vi "Convert to Waveforms.vi"(0 "data in":sgl[][](array[numeric]) format="%#.21g", 1 "physical channels":T1[](array[typedef])=[enum."Voltage Phase A (L1)", enum."Voltage Phase B (L2)", enum."Voltage Phase C (L3)", enum."Current Phase A (L1)", enum."Current Phase B (L2)", enum."Current Phase C (L3)", enum."Current Phase N (Neutral)"], 2 "reset? (F)":bool, 5 "sample rate [Hz]":sgl=9600.0 format="%#.6g", 7 "timestamp":timestamp, 9 "system info in":refnum<class "EP System Info.lvclass">, 11 "error in (no error)":errorcluster) -> (4 "voltage waveforms":waveform(dbl)[](array[waveform]), 6 "current waveforms":waveform(dbl)[](array[waveform]), 10 "system info out":refnum<class "EP System Info.lvclass">, 14 "interval length [s]":dbl, 15 "error out":errorcluster)   [LabVIEW 2014, in "NI_EP_Power Quality.lvlib"]
doc: "Converts resampled voltage and current data to voltage and current waveforms of different line configurations. This VI also arranges the order of the elements in the waveforms of each three-phase electrical power system for further measurement. For example, the orders are A-B-C-N for the four-channel method and A-B-C for the three-channel method. You must manually select the polymorphic instance you want to use."
uses:
  <vilib>/addons/Electrical Power/PQ/NI_EP_Power Quality.lvlib
  <vilib>/addons/Electrical Power/PQ/Common/Classes/System Info/EP System Info.lvclass
  <vilib>/addons/Electrical Power/PQ/Common/Controls/ep_AI Data Channel.ctl
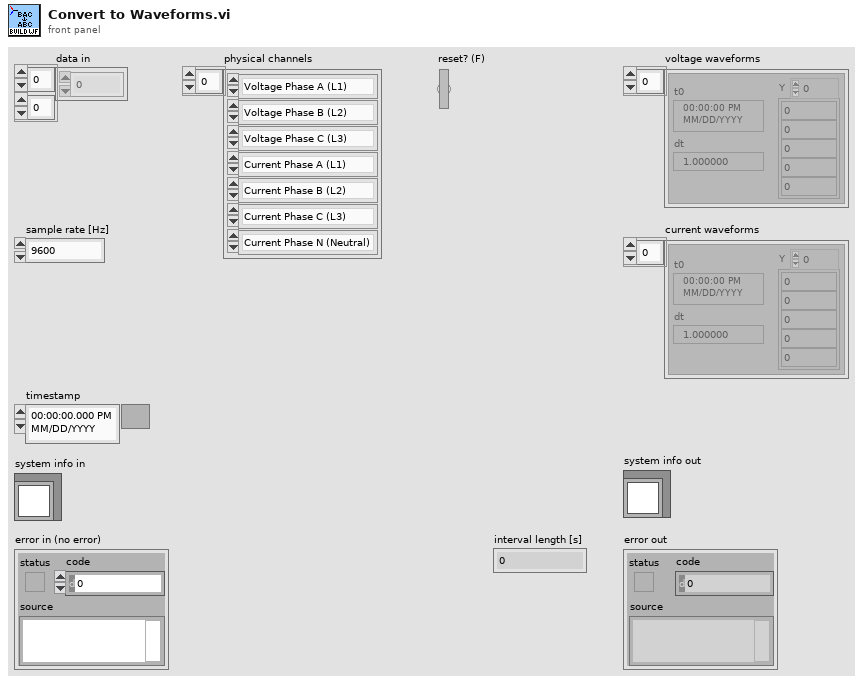
[diagram p1: front panel]
types:
  T1 = typedef "NI_EP_Power Quality.lvlib/ep_AI Data Channel.ctl" = enum16{"Voltage Phase A (L1)", "Voltage Phase B (L2)", "Voltage Phase C (L3)", "Voltage Phase N (Neutral)", "Current Phase A (L1)", "Current Phase B (L2)", "Current Phase C (L3)", "Current Phase N (Neutral)"}
  T2 = typedef "NI_EP_Power Quality.lvlib/ep_Wiring.ctl" = enum16{"4xUph + 4xI", "3xUph + 4xI", "3xUline + 4xI", "3xUph + 3xI", "3xUline + 3xI", "3xUph + 2xI", "3xUline + 2xI", "1xUph + 1xI"}
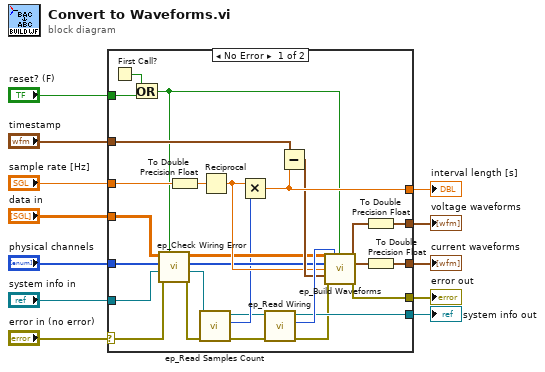
[diagram p0: block diagram]
diagram:
  n1 = case shown="No Error" "error in (no error)" {
    selector: "error in (no error)" -> [w29 w42]
    tunnel: "sample rate [Hz]" -> [w40 _]
    tunnel: "timestamp" -> [w39 _]
    tunnel: [w38 _] -> w10
    tunnel: [w14 _] -> w9
    tunnel: [w13 _] -> w8
    tunnel: "data in" -> [w26 _]
    tunnel: "physical channels" -> [w28 _]
    tunnel: [w34 w42] -> w5
    tunnel: [w16 w41] -> w4
    tunnel: "reset? (F)" -> [w23 _]
    tunnel: "system info in" -> [w24 w41]
    frame No Error {
      n2 = First Call?() -> (First Call?: T/F=w30:bool)
      n3 = Or(x=w30, y=w23) -> (x .or. y?=w22:bool)
      n4 = call <vilib>:"ep_Check Wiring Error.vi"("reset? (F)"=w22, "error in (no error)"=w29, "system info in"=w24, "physical channels in"=w28, "data in"=w26) -> ("error out"=w20:errorcluster, "system info out"=w21:refnum<class "EP System Info.lvclass">, "physical channels out"=w27:T1[], "data out"=w25:sgl[][])  [unwired: 3 in]
      n5 = To Double Precision Float(number=w40) -> (double precision float=w33:dbl)
      n6 = call <vilib>:"ep_Read Samples Count.vi"("error in (no error)"=w20, "system info in"=w21) -> ("error out"=w19:errorcluster, "basic calc. interval (samples)"=w18:i32, "system info out"=w17:refnum<class "EP System Info.lvclass">)  [unwired: 5 in, 2 out]
      n7 = Reciprocal(x=w33) -> (1/x=w31:dbl)
      n8 = Multiply(x=w31, y=w18) -> (x*y=w38:dbl)
      n9 = call <vilib>:"ep_Read Wiring.vi"("error in (no error)"=w19, "system info in"=w17) -> ("error out"=w15:errorcluster, "wiring"=w35:T2, "system info out"=w16:refnum<class "EP System Info.lvclass">)  [unwired: 6 in, 1 out]
      n10 = Subtract(x=w39, y=w38) -> (x-y=w32:timestamp)
      n11 = call <vilib>:"ep_Build Waveforms.vi"("AI data"=w25, "wiring"=w35, "reset? (F)"=w22, "AI data channel order"=w27, "dt"=w31, "t0"=w32, "error in (no error)"=w15) -> ("voltage waveforms"=w37:waveform(sgl)[], "current waveforms"=w36:waveform(sgl)[], "error out"=w34:errorcluster)  [unwired: 6 in]
      n12 = To Double Precision Float(number=w37) -> (double precision float=w14:waveform(dbl)[])
      n13 = To Double Precision Float(number=w36) -> (double precision float=w13:waveform(dbl)[])
    }
    frame Error {
    }
  }
  "voltage waveforms" <- w9
  "error out" <- w5
  "current waveforms" <- w8
  "system info out" <- w4
  "interval length [s]" <- w10
